vi "Set Channel Value by Data Reference.vi"(8 "error in":errorcluster, 9 "Value":dbl, 10 "Data Reference in":i32, 11 "NIVS Custom Device API in":refnum<class "NIVS Custom Device API.lvclass">) -> (0 "error out":errorcluster, 3 "NIVS Custom Device API out":refnum<class "NIVS Custom Device API.lvclass">)   [LabVIEW 2026, in "SystemMonitor Engine.lvlib" / "NIVS Custom Device API.lvclass"]
uses:
  NIVS Custom Device API.lvclass
  NIVS Custom Device API.lvclass/NIVS Custom Device API.ctl
  <vilib>/NI VeriStand/Custom Device API/Custom Device API.lvlib
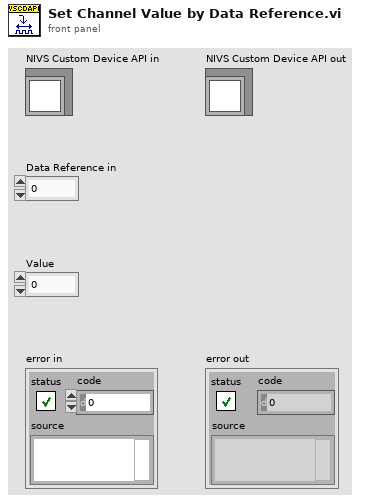
[diagram p1: front panel]
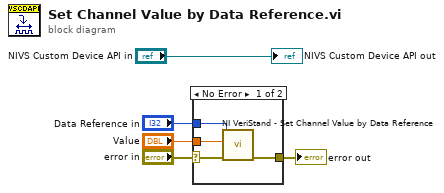
[diagram p0: block diagram]
diagram:
  n1 = case shown="No Error" "error in" {
    selector: "error in" -> [w9 w10]
    tunnel: [w8 w10] -> w3
    tunnel: "Data Reference in" -> [w7 _]
    tunnel: "Value" -> [w6 _]
    frame No Error {
      n2 = call <vilib>:"NI VeriStand - Set Channel Value by Data Reference.vi"("error in (no error)"=w9, "Value"=w6, "Data Reference in"=w7) -> ("error out"=w8:errorcluster)  [unwired: 8 in]
    }
    frame Error {
    }
  }
  "error out" <- w3
  "NIVS Custom Device API out" <- "NIVS Custom Device API in"
